vi "Song Generator Something uhhh.vi"() -> ()   [LabVIEW 2014]
uses:
  <vilib>/Utility/config.llb/NI_LVConfig.lvlib
panel:
  in  "configuration file path":path
  in  "Song":T1(array[cluster])=[{"frequency (Hz)"=328, "duration (msec)"=1000}, {"frequency (Hz)"=292, "duration (msec)"=1000}, {"frequency (Hz)"=261, "duration (msec)"=1000}, {"frequency (Hz)"=294, "duration (msec)"=1000}, {"frequency (Hz)"=332, "duration (msec)"=507}, {"frequency (Hz)"=332, "duration (msec)"=489}, {"frequency (Hz)"=328, "duration (msec)"=508}] {"duration (msec)" scale=200.0..1000.0; "frequency (Hz)" scale=261.0..523.0}
  in  "Load":bool
  in  "Save":bool
  in  "Play":bool
  # "C\nB\nA\nG\nF\nE\nD\nC"
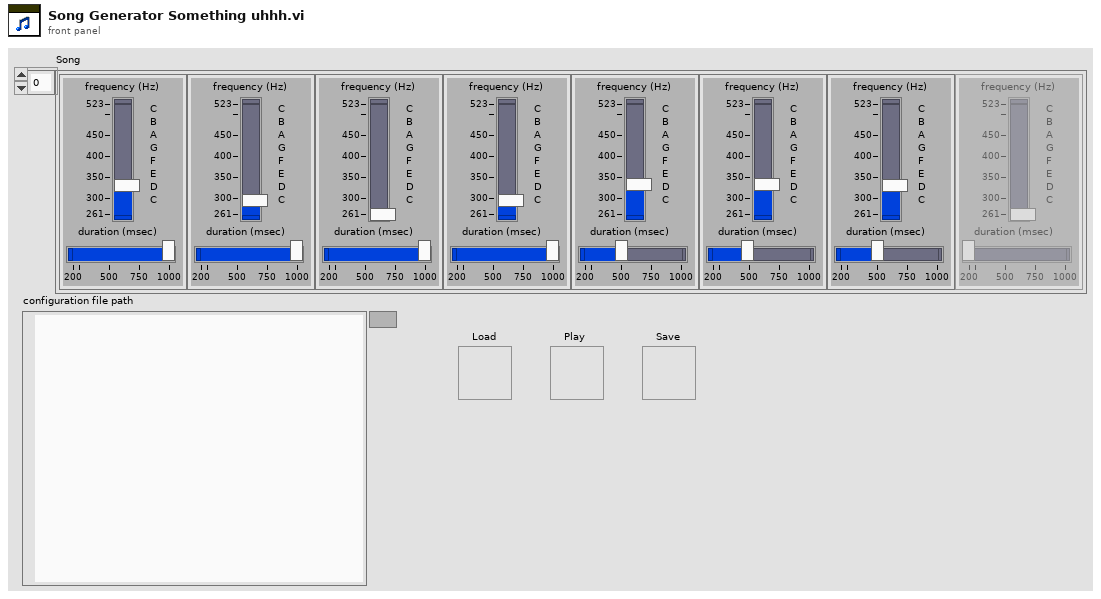
[diagram p1: front panel]
types:
  T1 = cluster{"frequency (Hz)":u32, "duration (msec)":u32}[]
  T2 = typedef "NI_LVConfig.lvlib/Config Data RefNum.ctl" = refnum<k1>
  T3 = cluster{"frequency (Hz)":u32, "duration (msec)":u32}
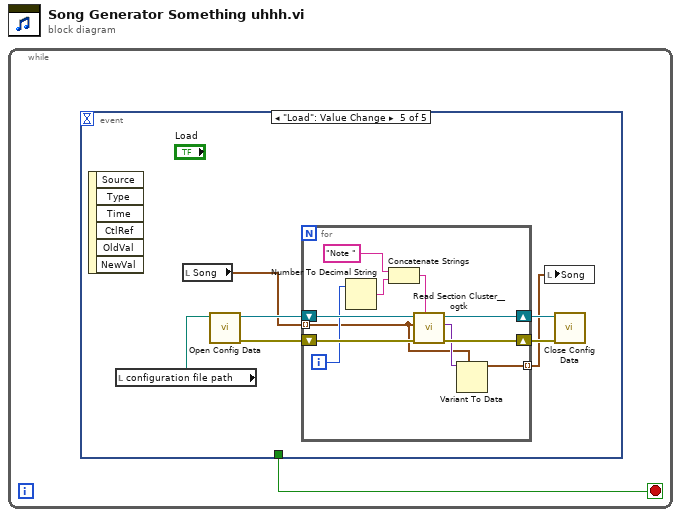
[diagram p0: block diagram]
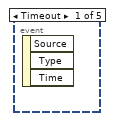
[diagram p2: hidden frame]
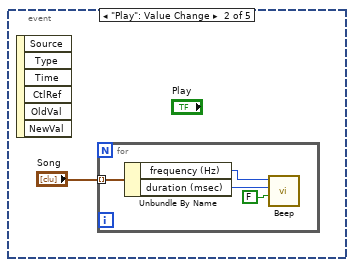
[diagram p3: hidden frame]
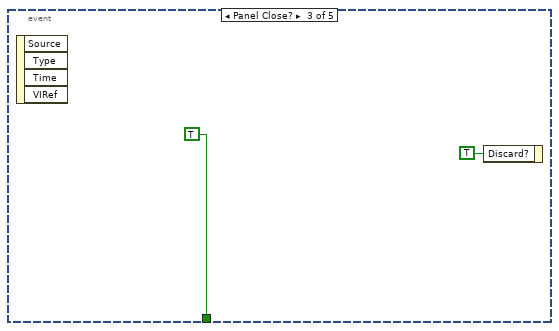
[diagram p4: hidden frame]
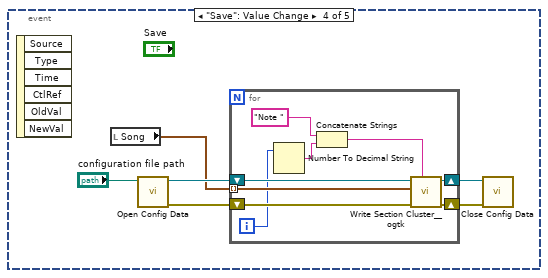
[diagram p5: hidden frame]
diagram:
  n1 = while {
    stop <- w1 stop-if-true
    n2 = event shown="[4] \"Load\": Value Change" {
      selector: _ -> [_ _ _ _ _]
      dyn-events: _ -> [_ _ _ _ _]
      timeout: _ -> [_ _ _ _ _]
      tunnel: [_ _ TRUE _ _] -> w1
      event Timeout {
        n3 = event-data() -> ()  [unwired: 1 in, 3 out]
      }
      event "Play": Value Change {
        n4 = event-data() -> ()  [unwired: 1 in, 6 out]
        n5 = for {
          tunnel: "Song" -> [w5] mode=indexing
          n6 = Unbundle By Name(w5) -> ("frequency (Hz)"=w4:u32, "duration (msec)"=w3:u32)
          n7 = call <vilib>:"Beep.vi"("use system alert? (T)"=FALSE, "duration (msec)"=w3, "frequency (Hz)"=w4) -> ()  [unwired: 9 in]
        }
      }
      event Panel Close? {
        n8 = event-data() -> ()  [unwired: 1 in, 4 out]
        n9 = event-data("Discard?"=TRUE) -> ()  [unwired: 1 in, 1 out]
      }
      event "Save": Value Change {
        n10 = event-data() -> ()  [unwired: 1 in, 6 out]
        n11 = local read "Song"() -> (w9:T1)
        n12 = call <vilib>:"Open Config Data.vi"("configuration file path"="configuration file path") -> ("error out"=w14:errorcluster, "refnum"=w12:T2)  [unwired: 8 in, 1 out]
        n13 = for {
          tunnel: w9 -> [w19] mode=indexing
          shift-right: [w22] -> w13
          shift-left: w14 -> [w23]
          shift-right: [w20] -> w11
          shift-left: w12 -> [w21]
          i -> [w18]
          n14 = Number To Decimal String(number=w18) -> (decimal integer string=w17:string)  [unwired: 1 in]
          n15 = Concatenate Strings("Note " ("section (optional)"), w17) -> (w15:string)
          n16 = call <userlib>:"Write Section Cluster__ogtk.vi"("section (optional)"=w15, "error in (no error)"=w23, "Section Formatted Cluster"=w19, "refnum"=w21) -> ("error out"=w22:errorcluster, "dup refnum"=w20:T2)  [unwired: 6 in]
        }
        n17 = call <vilib>:"Close Config Data.vi"("error in (no error)"=w13, "refnum"=w11) -> ()  [unwired: 8 in, 2 out]
      }
      event "Load": Value Change {
        n18 = event-data() -> ()  [unwired: 1 in, 6 out]
        n19 = local read "configuration file path"() -> (w25:path)
        n20 = local read "Song"() -> (w26:T1)
        n21 = call <vilib>:"Open Config Data.vi"("configuration file path"=w25) -> ("error out"=w30:errorcluster, "refnum"=w28:T2)  [unwired: 8 in, 1 out]
        n22 = for {
          tunnel: w26 -> [w32] mode=indexing
          shift-right: [w40] -> w29
          shift-left: w30 -> [w41]
          shift-right: [w38] -> w27
          shift-left: w28 -> [w39]
          tunnel: [w31] -> w24 mode=indexing
          i -> [w37]
          n23 = Number To Decimal String(number=w37) -> (decimal integer string=w36:string)  [unwired: 1 in]
          n24 = Concatenate Strings("Note " ("section (optional)"), w36) -> (w34:string)
          n25 = call <userlib>:"Read Section Cluster__ogtk.vi"("section (optional)"=w34, "error in (no error)"=w41, "Section Formatted Cluster Type"=w32, "refnum"=w39) -> ("error out"=w40:errorcluster, "Section Formatted Cluster"=w33:variant, "dup refnum"=w38:T2)  [unwired: 3 in, 2 out]
          n26 = Variant To Data(type=w32, Variant=w33) -> (data=w31:T3)  [unwired: 1 in, 1 out]
        }
        n27 = local write "Song"(w24) -> ()
        n28 = call <vilib>:"Close Config Data.vi"("error in (no error)"=w29, "refnum"=w27) -> ()  [unwired: 8 in, 2 out]
      }
    }
  }
